vi "Inst_CNT90.vi"(8 "error in":errorcluster, 10 "All Message Queues in":T1, 11 "Prueba31 in":refnum<class "Prueba08.lvclass">) -> (0 "error out":errorcluster)   [LabVIEW 2019, in "Prueba08.lvclass"]
uses:
  Prueba08.lvclass
  QMH/Message Queue/All Message Queues.ctl
  QMH/Message Queue/Message Cluster.ctl
  Prueba08.lvclass/Prueba08.ctl
  <vilib>/Utility/error.llb/Error Cluster From Error Code.vi
  QMH/Message Queue/Enqueue Message (Single).vi
  <vilib>/ErrorRing/Error Ring.xnode
  QMH/Message Queue/Message Queue.lvlib
  Instrumento/CNT90/CNT90.lvclass
panel:
  out "All States":string[](array[string])
  out "Actual State":string
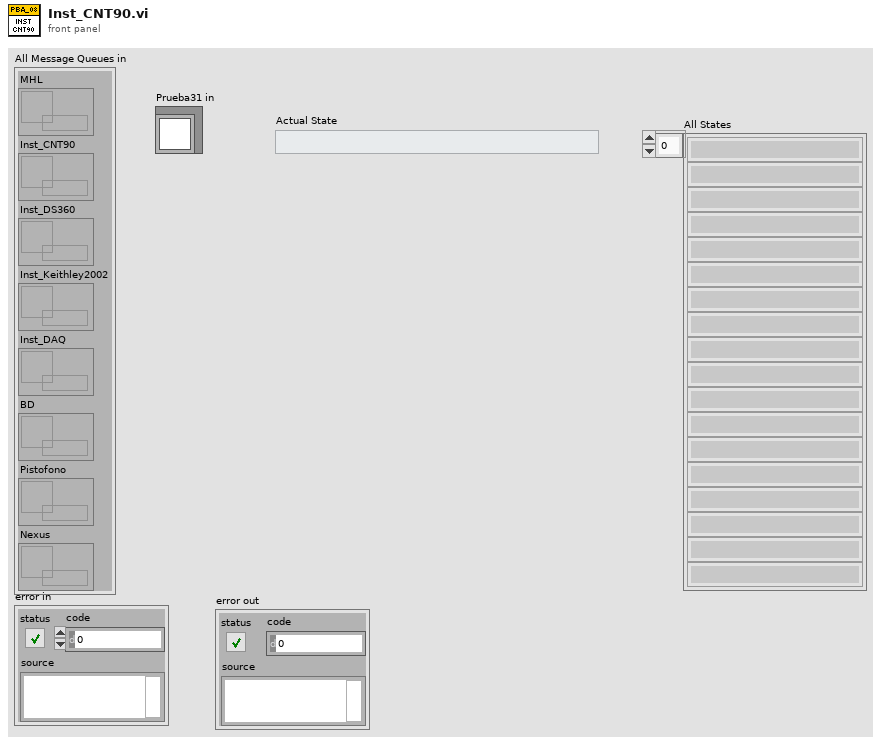
[diagram p1: front panel]
types:
  T1 = typedef "Message Queue.lvlib/All Message Queues.ctl" = cluster{"MHL":refnum<queue>, "Inst_CNT90":refnum<queue>, "Inst_DS360":refnum<queue>, "Inst_Keithley2002":refnum<queue>, "Inst_DAQ":refnum<queue>, "BD":refnum<queue>, "Pistofono":refnum<queue>, "Nexus":refnum<queue>}
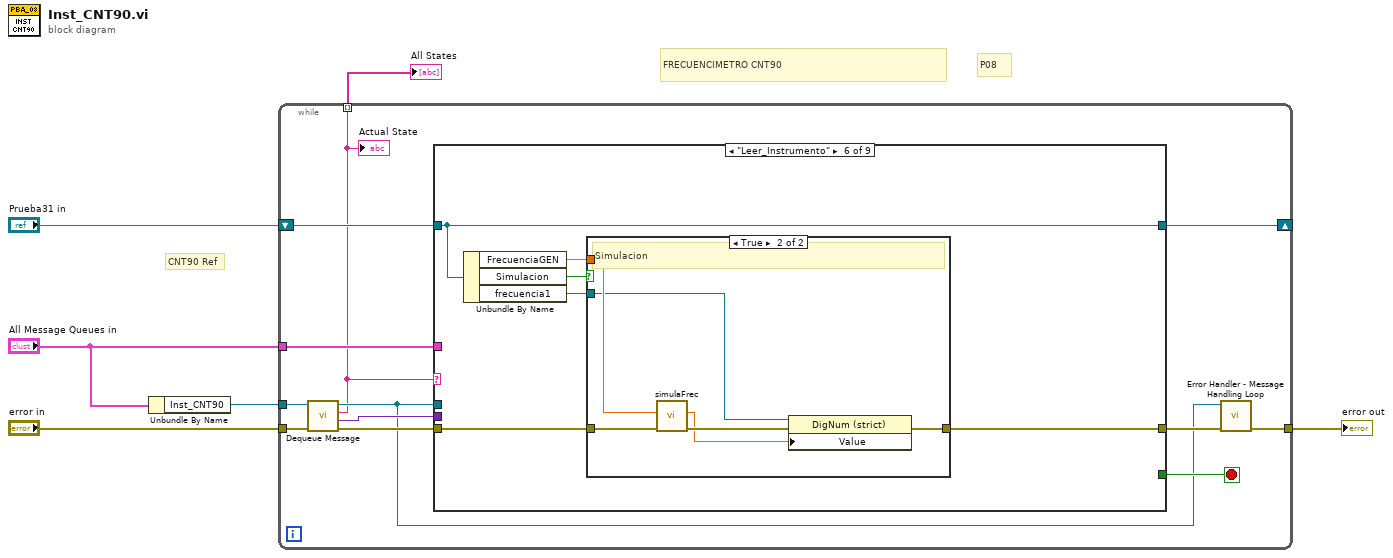
[diagram p0: block diagram]
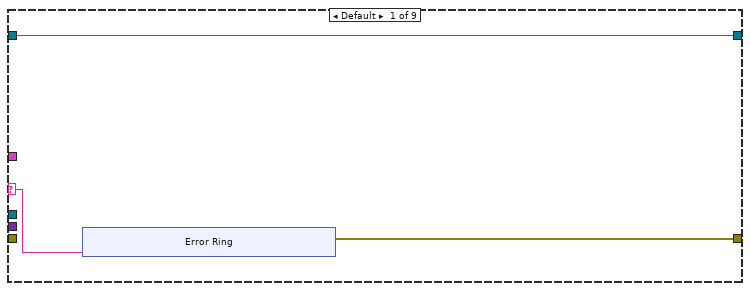
[diagram p2: hidden frame]
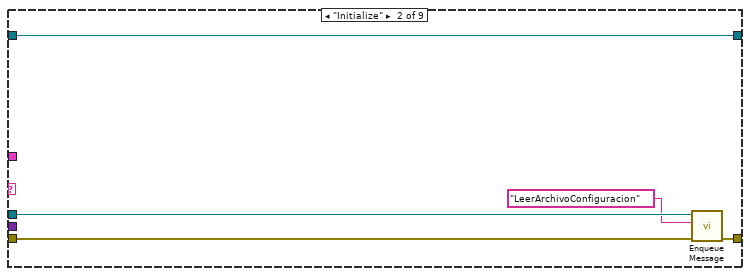
[diagram p3: hidden frame]
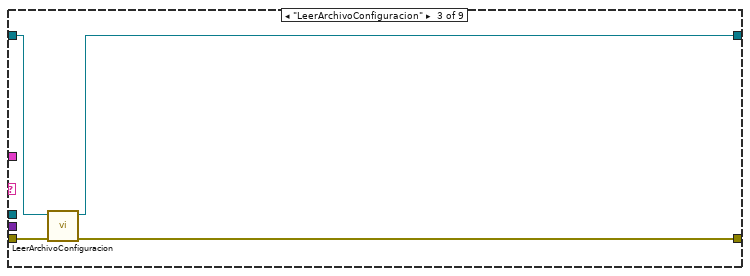
[diagram p4: hidden frame]
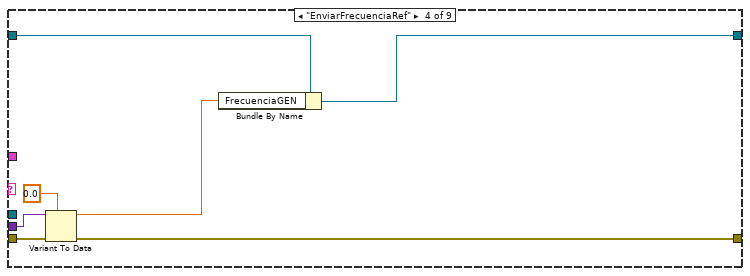
[diagram p5: hidden frame]
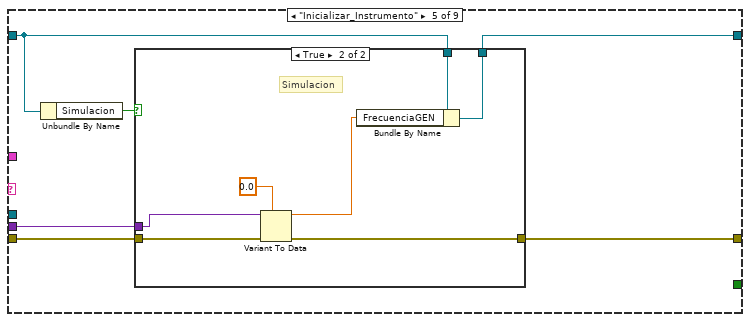
[diagram p6: hidden frame]
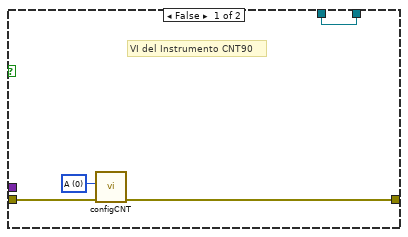
[diagram p7: hidden frame]
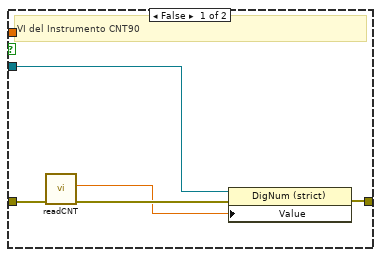
[diagram p8: hidden frame]
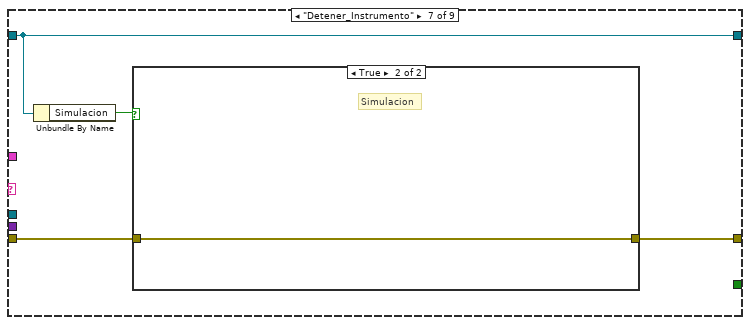
[diagram p9: hidden frame]
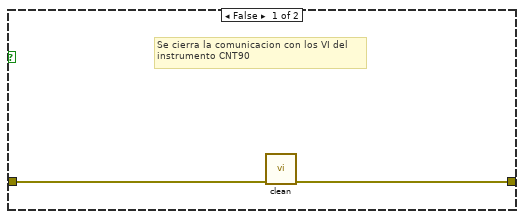
[diagram p10: hidden frame]
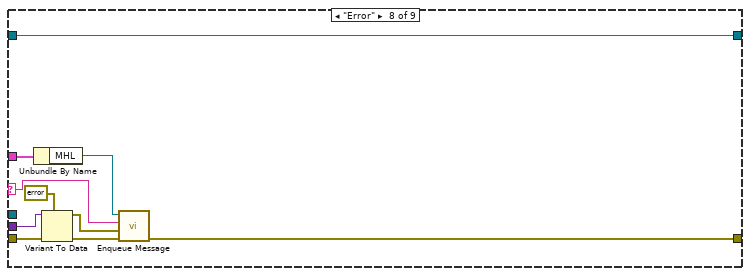
[diagram p11: hidden frame]
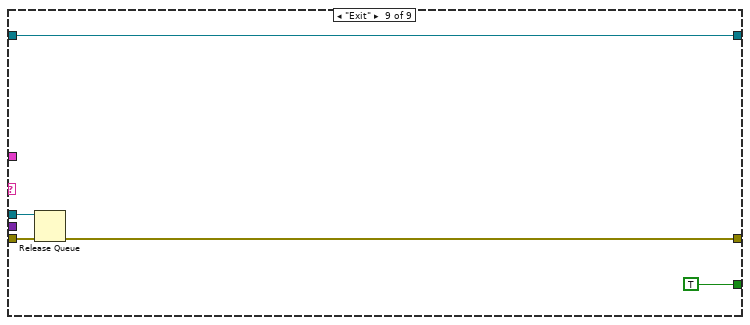
[diagram p12: hidden frame]
diagram:
  # "P08"
  # "FRECUENCIMETRO CNT90"
  # "CNT90 Ref"
  n1 = Unbundle By Name("All Message Queues in") -> ("Inst_CNT90"=w4:refnum<queue>)
  n2 = while {
    tunnel: "error in" -> [w18]
    tunnel: w4 -> [w17]
    tunnel: "All Message Queues in" -> [w16]
    tunnel: [w9] -> w2
    shift-right: [w12] -> _
    shift-left: "Prueba31 in" -> [w15]
    tunnel: [w7] -> w1 mode=indexing
    stop <- w11 stop-if-true
    n3 = call "Dequeue Message.vi"("error in (no error)"=w18, "Message Queue"=w17) -> ("error out"=w13:errorcluster, "Message Data"=w14:variant, "Message"=w7:string, "dup Message Queue"=w8:refnum<queue>)  [unwired: 6 in]
    "Actual State" <- w7
    n4 = case shown="\"Leer_Instrumento\"" w7 {
      selector: w7 -> [w21 _ _ _ _ _ _ w90 _]
      tunnel: w16 -> [_ _ _ _ _ _ _ w89 _]
      tunnel: w15 -> [w19 w33 w34 w39 w46 w66 w81 w87 w97]
      tunnel: w8 -> [_ w30 _ _ _ _ _ _ w99]
      tunnel: w14 -> [_ _ _ w42 w47 _ _ w93 _]
      tunnel: w13 -> [_ w31 w35 w43 w50 w67 w79 w94 w100]
      tunnel: [w20 w32 w37 w44 w48 w62 w82 w86 w96] -> w10
      tunnel: [w19 w33 w36 w40 w45 w66 w81 w87 w97] -> w12
      tunnel: [_ _ _ _ _ _ _ _ TRUE] -> w11
      frame Default {
        n5 = xnode "Error Ring"("parameter 0"=w21) -> ("error out"=w20:errorcluster)
      }
      frame "Initialize" {
        n6 = call-poly "Enqueue Message.vi"("error in (no error)"=w31, "Message"="LeerArchivoConfiguracion", "Message Queue"=w30) -> ("error out"=w32:errorcluster)  [unwired: 7 in, 1 out]
      }
      frame "LeerArchivoConfiguracion" {
        n7 = call "LeerArchivoConfiguracion.vi"("error in"=w35, "Prueba31 in"=w34) -> ("error out"=w37:errorcluster, "Prueba31 out"=w36:refnum<class "Prueba08.lvclass">)  [unwired: 8 in]
      }
      frame "EnviarFrecuenciaRef" {
        n8 = Variant To Data(error in=w43, type=0.0, Variant=w42) -> (data=w38:dbl, error out=w44:errorcluster)
        n9 = Bundle By Name(cluster=w39, "FrecuenciaGEN"=w38) -> (w40:refnum<class "Prueba08.lvclass">)
      }
      frame "Inicializar_Instrumento" {
        n10 = Unbundle By Name(w46) -> ("Simulacion"=w49:bool)
        n11 = case shown="True" w49 {
          tunnel: [w54 w60] -> w48
          tunnel: w50 -> [w53 w61]
          tunnel: w47 -> [_ w59]
          tunnel: w46 -> [w51 w57]
          tunnel: [w51 w56] -> w45
          frame False {
            w52 = 0 items=["A", "B"] ("Channel  1")
            # "VI del Instrumento CNT90"
            n12 = call "configCNT.vi"("error in (no error)"=w53, "Channel  1"=w52) -> ("error out"=w54:errorcluster)  [unwired: 8 in, 1 out]
          }
          frame True {
            # "Simulacion"
            n13 = Variant To Data(error in=w61, type=0.0, Variant=w59) -> (data=w55:dbl, error out=w60:errorcluster)
            n14 = Bundle By Name(cluster=w57, "FrecuenciaGEN"=w55) -> (w56:refnum<class "Prueba08.lvclass">)
          }
        }
      }
      frame "Leer_Instrumento" {
        n15 = Unbundle By Name(w66) -> ("FrecuenciaGEN"=w64:dbl, "Simulacion"=w65:bool, "frecuencia1"=w63:refnum<vi>)
        n16 = case shown="True" w65 {
          tunnel: w67 -> [w72 w78]
          tunnel: w64 -> [_ w77]
          tunnel: w63 -> [w71 w76]
          tunnel: [w69 w73] -> w62
          frame False {
            # "VI del Instrumento CNT90"
            n17 = call "readCNT.vi"("error in (no error)"=w72) -> ("error out"=w70:errorcluster, "medicion"=w68:dbl)  [unwired: 8 in, 1 out]
            n18 = property class="DigNum (strict)"(reference=w71, error in=w70, "Value"=w68) -> (error out=w69:errorcluster)  [unwired: 1 out]
          }
          frame True {
            # "Simulacion"
            n19 = call "simulaFrec.vi"("error in (no error)"=w78, "frec in"=w77) -> ("error out"=w75:errorcluster, "frec out"=w74:dbl)  [unwired: 7 in, 1 out]
            n20 = property class="DigNum (strict)"(reference=w76, error in=w75, "Value"=w74) -> (error out=w73:errorcluster)  [unwired: 1 out]
          }
        }
      }
      frame "Detener_Instrumento" {
        n21 = Unbundle By Name(w81) -> ("Simulacion"=w80:bool)
        n22 = case shown="True" w80 {
          tunnel: [w84 w85] -> w82
          tunnel: w79 -> [w83 w85]
          frame False {
            # "Se cierra la comunicacion con los VI del\ninstrumento CNT90"
            n23 = call "clean.vi"("error in (no error)"=w83) -> ("error out"=w84:errorcluster)  [unwired: 9 in, 1 out]
          }
          frame True {
            # "Simulacion"
          }
        }
      }
      frame "Error" {
        n24 = Unbundle By Name(w89) -> ("MHL"=w88:refnum<queue>)
        n25 = Variant To Data(error in=w94, type=errorcluster {"status"=FALSE, "code"=0, "source"=""} ("error constant"), Variant=w93) -> (data=w91:errorcluster, error out=w92:errorcluster)
        n26 = call-poly "Enqueue Message.vi"("error in (no error)"=w92, "Message Data"=w91, "Message"=w90, "Message Queue"=w88) -> ("error out"=w86:errorcluster)  [unwired: 6 in, 1 out]
      }
      frame "Exit" {
        n27 = Release Queue(queue=w99, error in (no error)=w100) -> (error out=w96:errorcluster)  [unwired: 1 in, 2 out]
      }
    }
    n28 = call "Error Handler - Message Handling Loop.vi"("error in (no error)"=w10, "Message Queue"=w8) -> ("dup error in"=w9:errorcluster)  [unwired: 8 in, 1 out]
  }
  "error out" <- w2
  "All States" <- w1
